vi "Actor Core.vi"(8 "error in":errorcluster, 11 "Server in":refnum<class "Server.lvclass">) -> (0 "error out":errorcluster, 3 "Actor out":refnum<class "Actor.lvclass">)   [LabVIEW 2020, in "Server.lvlib" / "Server.lvclass"]
doc: "(<B>Filename</B>: Actor Framework.lvlib:Actor.lvclass:Actor Core.vi)\n\nReceives messages to the actor, reacts to them, and initiates any error handling that may shut the actor down.\n\nDescendant classes may override this VI to append parallel tasks for the actor to complete while it handles messages. Overrides use the Call Parent Class Method node."
uses:
  Server.lvclass
  C:/Program Files (x86)/National Instruments/LabVIEW 2020/vi.lib/ActorFramework/Actor/Actor.lvclass
  <vilib>/ActorFramework/Actor/Actor.lvclass
  <vilib>/ActorFramework/Actor/Actor.lvclass/Actor.ctl
  <vilib>/ActorFramework/Message Enqueuer/Message Enqueuer.lvclass/Message Enqueuer.ctl
  Server.lvclass/Server.ctl
  Server Messages/Global Chat Msg/Global Chat Msg.lvclass/Global Chat Msg.ctl
  <vilib>/ActorFramework/Message Enqueuer/Init from Existing Queue.vi
  <vilib>/ActorFramework/Message Enqueuer/Enqueue.vi
  Server Messages/Lanuch New Chat Window Msg/Lanuch New Chat Window Msg.lvclass
  C:/Program Files (x86)/National Instruments/LabVIEW 2020/vi.lib/ActorFramework/Message/Message.lvclass
  Server Messages/Global Chat Msg/Global Chat Msg.lvclass
  <vilib>/ActorFramework/Stop Msg/Stop Msg.lvclass
  <vilib>/ActorFramework/Message Priority Queue/Priority Enqueue.vi
  <vilib>/ActorFramework/Message Enqueuer/Message Enqueuer.lvclass
panel:
  in  "Send Global Chat":bool
  in  "Launch Chat Window":bool
  in  "Global Message":string
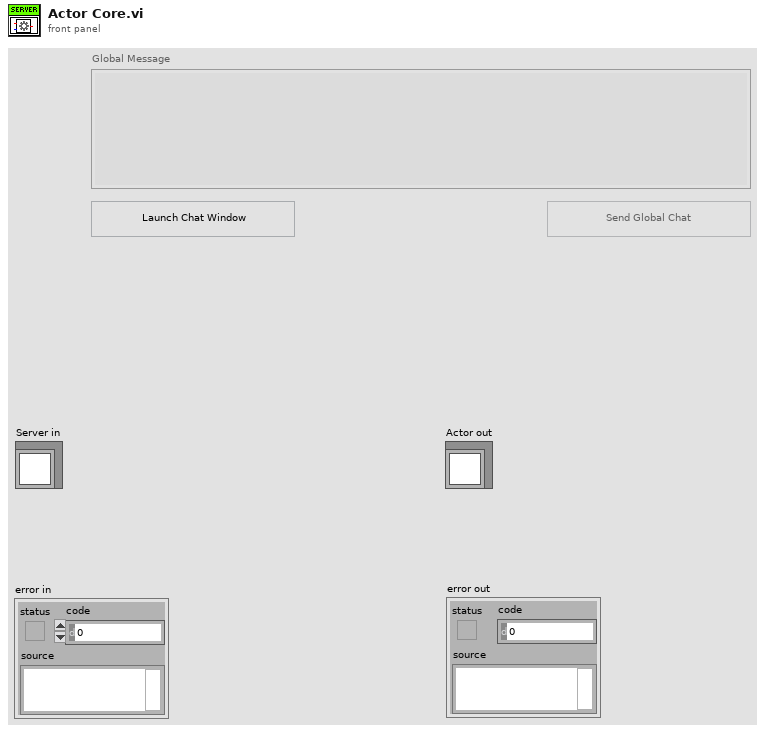
[diagram p1: front panel]
types:
  T1 = enum8{"Enabled", "Disabled", "Disabled and Grayed Out"}
  T2 = enum32{"Invalid", "Standard", "Closed", "Hidden", "Minimized", "Maximized"}
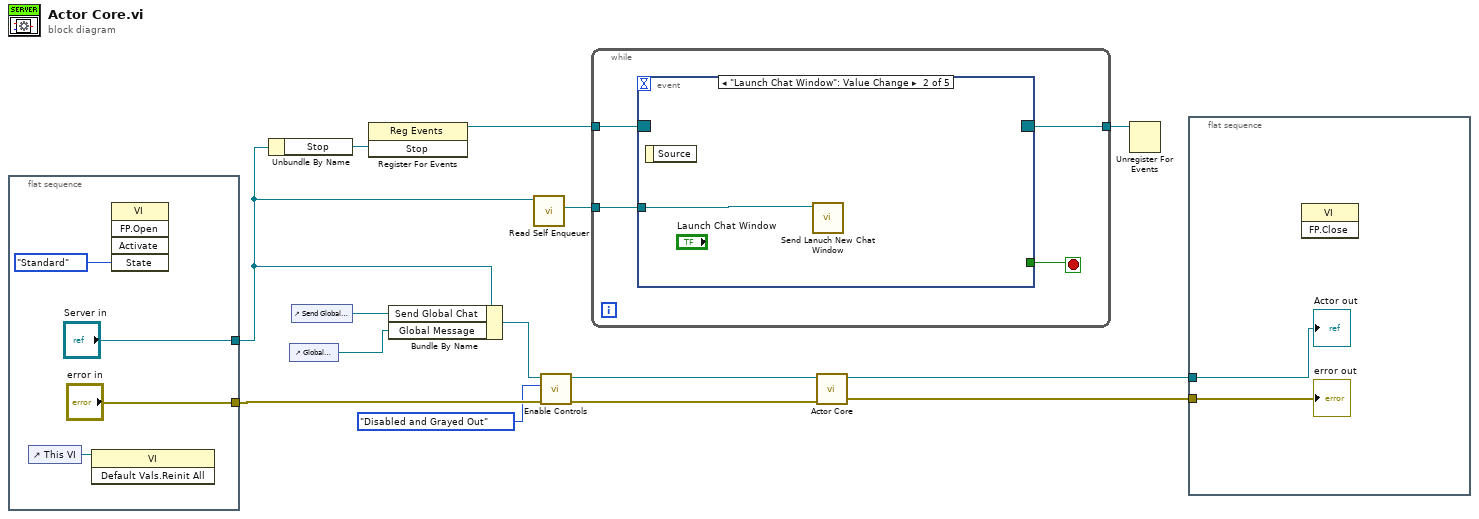
[diagram p0: block diagram]
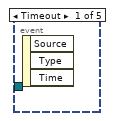
[diagram p2: hidden frame]
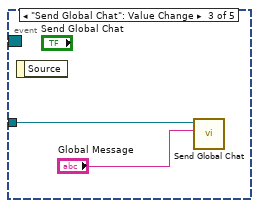
[diagram p3: hidden frame]
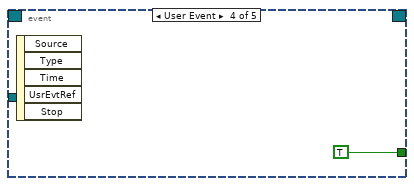
[diagram p4: hidden frame]
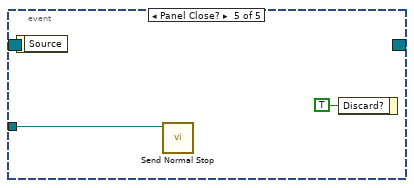
[diagram p5: hidden frame]
diagram:
  n1 = flat-sequence {
    tunnel: ["error in"] -> w7
    tunnel: ["Server in"] -> w4
    frame #0 {
      n2 = control-ref of="This VI"() -> (w15:refnum<vi>)
      n3 = invoke class="VI" method="Default Vals.Reinit All"(reference=w15) -> ()  [unwired: 2 in, 3 out]
      n4 = invoke class="VI" method="FP.Open"("State"=T2."Standard") -> ()  [unwired: 4 in, 5 out]
    }
  }
  n5 = Unbundle By Name(w4) -> ("Stop"=w11:refnum<user-event>)
  n6 = control-ref of="Global Message"() -> (w2:refnum<vi>)
  n7 = control-ref of="Send Global Chat"() -> (w3:refnum<vi>)
  n8 = register-events(w11) -> (reference out=w10:refnum<event-registration>)  [unwired: 2 in, 1 out]
  n9 = Bundle By Name(cluster=w4, "Send Global Chat"=w3, "Global Message"=w2) -> (w1:refnum<class "Server.lvclass">)
  n10 = call <vilib>:"Read Self Enqueuer.vi"("Actor"=w4) -> ("Self Enqueuer"=w12:refnum<class "Message Enqueuer.lvclass">)  [unwired: 10 in]
  n11 = call "Enable Controls.vi"("error in (no error)"=w7, "Disabled"=T1."Disabled and Grayed Out", "Server in"=w1) -> ("error out"=w6:errorcluster, "Server out"=w8:refnum<class "Server.lvclass">)  [unwired: 7 in]
  n12 = while {
    tunnel: w12 -> [w22]
    tunnel: w10 -> [w21]
    tunnel: [w20] -> w9
    stop <- w19 stop-if-true
    n13 = event shown="[1] \"Launch Chat Window\": Value Change" {
      selector: w21 -> [_ _ _ _ _]
      dyn-events: [_ _ _ _ _] -> w20
      timeout: _ -> [_ _ _ _ _]
      tunnel: w22 -> [_ w23 w25 _ w27]
      tunnel: [_ _ _ TRUE _] -> w19
      event Timeout {
        n14 = event-data() -> ()  [unwired: 1 in, 3 out]
      }
      event "Launch Chat Window": Value Change {
        n15 = event-data() -> ()  [unwired: 1 in, 1 out]
        n16 = call "Send Lanuch New Chat Window.vi"("Message Enqueuer"=w23) -> ()  [unwired: 9 in, 2 out]
      }
      event "Send Global Chat": Value Change {
        n17 = event-data() -> ()  [unwired: 1 in, 1 out]
        n18 = call "Send Global Chat.vi"("Global Msg"="Global Message", "Message Enqueuer"=w25) -> ()  [unwired: 8 in, 2 out]
      }
      event User Event {
        n19 = event-data() -> ()  [unwired: 1 in, 5 out]
      }
      event Panel Close? {
        n20 = event-data() -> ()  [unwired: 1 in, 1 out]
        n21 = call <vilib>:"Send Normal Stop.vi"("Message Enqueuer"=w27) -> ()  [unwired: 10 in, 1 out]
        n22 = event-data("Discard?"=TRUE) -> ()  [unwired: 1 in, 1 out]
      }
    }
  }
  n23 = call-parent "Actor Core.vi"("error in"=w6, "Actor in"=w8) -> ("error out"=w14:errorcluster, "Actor out"=w13:refnum<class "Actor.lvclass">)  [unwired: 8 in]
  n24 = Unregister For Events(event registration refnum=w9) -> ()  [unwired: 1 in, 1 out]
  n25 = flat-sequence {
    tunnel: w14 -> [w30]
    tunnel: w13 -> [w29]
    frame #0 {
      n26 = invoke class="VI" method="FP.Close"() -> ()  [unwired: 3 in, 3 out]
      "error out" <- w30
      "Actor out" <- w29
    }
  }
